vi "Configure Waveform (Square).vi"(0 "VISA resource name":refnum<visa-resource-name>, 1 "Start Level (0)":dbl, 2 "Start Time (0 second)":dbl, 5 "Output Channel (0: Channel 1)":i32(ring) items=["Channel 1", "Channel 2"], 7 "Source Mode (1: Voltage)":i32(ring)=1 items=["Current", "Voltage"], 9 "Top Time (0 second)":dbl, 11 "error in (no error)":errorcluster, 12 "Top Level (0)":dbl, 13 "End Time (0 second)":dbl) -> (4 "VISA resource name out":refnum<visa-resource-name>, 15 "error out":errorcluster)   [LabVIEW 2020, in "Agilent B2900 Series.lvlib"]
doc: "Configure current or voltage square waveform output.\n\n<B>Note:</B>\nThis VI is only supported by Agilent models B2961A, B2962A, B2961B,B2962B,B2961C and B2962C."
uses:
  Agilent B2900 Series.lvlib
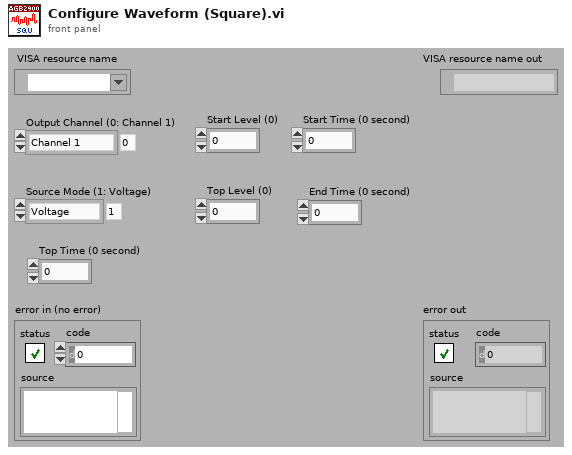
[diagram p1: front panel]
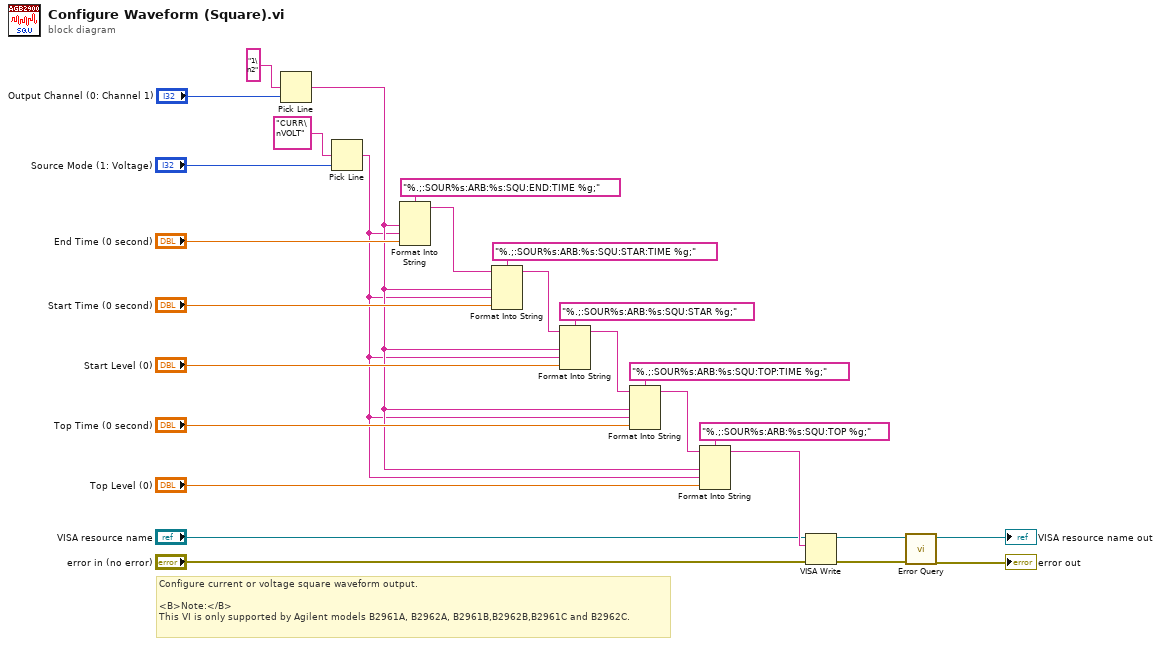
[diagram p0: block diagram]
diagram:
  # "Configure current or voltage square waveform output.\n\n<B>Note:</B>\nThis VI is only supported by Agilent models B2961A, B2962A, B2961B,B2962B,B2961C and B2962C."
  n1 = Pick Line(multi-line string="1\n2", line index="Output Channel (0: Channel 1)") -> (output string=w2:string)  [unwired: 1 in]
  n2 = Pick Line(multi-line string="CURR\nVOLT", line index="Source Mode (1: Voltage)") -> (output string=w1:string)  [unwired: 1 in]
  n3 = Format Into String(format string="%.;:SOUR%s:ARB:%s:SQU:END:TIME %g;", w2, w1, "End Time (0 second)") -> (resulting string=w26:string)  [unwired: 2 in, 1 out]
  n4 = Format Into String(format string="%.;:SOUR%s:ARB:%s:SQU:STAR:TIME %g;", initial string=w26, w2, w1, "Start Time (0 second)") -> (resulting string=w24:string)  [unwired: 1 in, 1 out]
  n5 = Format Into String(format string="%.;:SOUR%s:ARB:%s:SQU:STAR %g;", initial string=w24, w2, w1, "Start Level (0)") -> (resulting string=w21:string)  [unwired: 1 in, 1 out]
  n6 = Format Into String(format string="%.;:SOUR%s:ARB:%s:SQU:TOP:TIME %g;", initial string=w21, w2, w1, "Top Time (0 second)") -> (resulting string=w19:string)  [unwired: 1 in, 1 out]
  n7 = Format Into String(format string="%.;:SOUR%s:ARB:%s:SQU:TOP %g;", initial string=w19, w2, w1, "Top Level (0)") -> (resulting string=w17:string)  [unwired: 1 in, 1 out]
  n8 = VISA Write(VISA resource name="VISA resource name", write buffer=w17, error in (no error)="error in (no error)") -> (VISA resource name out=w14:refnum<visa-resource-name>, error out=w13:errorcluster)  [unwired: 1 out]
  n9 = call "Error Query.vi"("error in (no error)"=w13, "VISA resource name"=w14) -> ("error out"=→"error out":errorcluster, "VISA resource name out"=→"VISA resource name out":refnum<visa-resource-name>)  [unwired: 8 out]
